vi "Turret Controller.vi"(8 "error in":errorcluster) -> ()   [LabVIEW 2015]
doc: "This VI executes continuously carrying out the current operation and responding to updates or new operations. It will often contain the timing or control code that is difficult to place directly in TeleOp. This VI generally opens all sensors and motors and isolates the rest of the robot code from knowing how the operations are carried out."
uses:
  Turret Setpoints.ctl
  Turret Operations.ctl
  <vilib>/Rock Robotics/WPI/CAN/TalonSRX/WPI_CANTalonSRX_APIControlMode.ctl
  <vilib>/Rock Robotics/WPI/CAN/TalonSRX/WPI_CANTalonSRX_APIFeedbackSelect.ctl
  <vilib>/Rock Robotics/WPI/CAN/TalonSRX/WPI_CANTalonSRX_Params.ctl
  <vilib>/Rock Robotics/WPI/MotorControl/WPI_MotorControlOpenCANTalonSRX.vi
  Framework/Robot Global Data.vi
  Vision/Vision Published Globals.vi
  Turret Published Globals.vi
  Support Code/navX Library v2/navX Library v2.lvlib
panel:
  out "Current\nCmd":string
  # "Tip: It may be helpful to observe inputs and sensor values.\nYou may also want to display tuning or debugging controls."
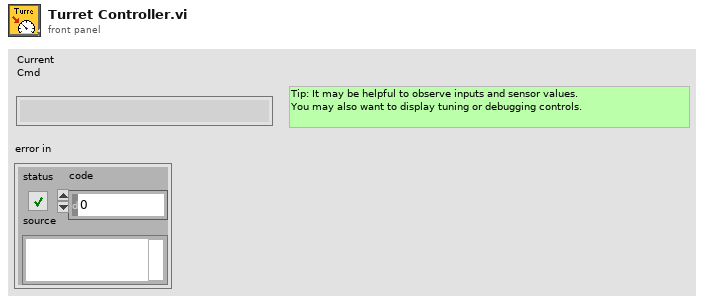
[diagram p1: front panel]
types:
  T1 = typedef "Turret Setpoints.ctl" = cluster{"Operation":T2, "Setpoint":dbl, "Duration":dbl}
  T2 = typedef "Turret Operations.ctl" = enum16{"Reserve", "Read Current", "Go to Angle (Turret Centric)", "Idle", "Go to Angle (Field Centric)", "Roaming", "Go to Angle", "Manual Control"}
  T3 = typedef "WPI_CANTalonSRX_APIFeedbackSelect.ctl" = enum16{"Digital Quadrature Encoder", "Analog Potentiometer", "Analog Encoder", "Count on Quad-A (Rising-Edge)", "Count on Quad-A (Falling-Edge)", "CTR Magnetic Enc (Absolute)", "CTR Magnetic Enc (Relative)", "Pulse Width"}
  T4 = typedef "WPI_CANTalonSRX_APIControlMode.ctl" = enum8{"Percent VBus", "Speed", "Position", "Slave", "Unchanged / Invalid", "Voltage Compensation", "Current", "Motion Profile"}
  T5 = typedef "WPI_MotorControlDeviceRef.ctl" = cluster{"DeviceStatus":errorcluster, "Type":T6, "PWM":cluster{"PWM Channel":T7, "DeadBand":T8}, "CAN":cluster{"Device Number":u8, "Control Mode":T9, "Semaphore":T10, "Max Vout":dbl, "TalonSRX Control Mode":T4}, "Invert":bool}
  T6 = typedef "WPI_MotorControlType.ctl" = enum16{"PWM", "CAN", "CANTalonSRX"}
  T7 = typedef "FPGA_DIOPWMChannel.ctl" = enum8{"PWM 0", "PWM 1", "PWM 2", "PWM 3", "PWM 4", "PWM 5", "PWM 6", "PWM 7", "PWM 8", "PWM 9", "PWM MXP 0", "PWM MXP 1", "PWM MXP 2", "PWM MXP 3", "PWM MXP 4", "PWM MXP 5", "PWM MXP 6", "PWM MXP 7", "PWM MXP 8", "PWM MXP 9", "Invalid"}
  T8 = typedef "WPI_PWMDeadband.ctl" = cluster{"Name":string, "maxPositivePwm":i32, "minPositivePwm":i32, "centerPwm":i32, "maxNegativePwm":i32, "minNegativePwm":i32, "angularRange":u16}
  T9 = typedef "WPI_CANJaguar_ControlMode.ctl" = enum8{"Percent VBus", "Current", "Speed", "Position", "Voltage"}
  T10 = typedef "Semaphore RefNum" = refnum<k1>
  T11 = typedef "navX Library v2.lvlib/Z900_navX_DeviceTypeDef.ctl" = cluster{"Interface":cluster{"Protocol":T12, "Update Rate (4Hz-60Hz)":u8, "navX Open TypeDef":variant}, "Notify Packet":refnum<notifier>, "Loop VI Refnum":refnum<vi>, "Ready to Close Occurrence Refnum":refnum<k4>}
  T12 = typedef "navX Library v2.lvlib/Z900_navX_ProtocolTypeDef.ctl" = enum16{"SERIAL", "I2C", "SPI"}
  T13 = typedef "WPI_CANTalonSRX_Params.ctl" = u8
  T14 = typedef "Command Status Info.ctl" = cluster{"Name":string, "Status":T15, "notifier out":T16}
  T15 = typedef "Completion Status.ctl" = enum16{"Successful", "Aborted", "Incomplete"}
  T16 = typedef "Completion Notifier.ctl" = refnum<notifier>
  T17 = cluster{"Default Command":T1, "Command Timing":cluster{"Start Time (ms)":u32, "Iterations":i32}, "Command Arguments":cluster{"Command Info":T14, "Description":string, "Default Command":T1, "notifier out":refnum<notifier>, "Subsystem Name":string}}
  T18 = cluster{"Yaw":dbl, "Roll":dbl, "Pitch":dbl, "Heading":dbl, "Fused Heading":dbl}
  T19 = typedef "WPI_CANTalonSRX_GlobalStatus.ctl" = cluster{"Applied Throttle":dbl, "Module Enabled":bool, "CAN Error":errorcluster, "Closed Loop Error":dbl, "Forward Limit Switch Closed":bool, "Reverse Limit Switch Closed":bool, "Sensor Position":dbl, "Sensor Velocity":dbl, "Current":dbl, "Sticky Fault - Over Temp":bool, "Sticky Fault - Under Voltage":bool, "Sticky Fault - Forward Limit":bool, "Sticky Fault - Reverse Limit":bool, "Sticky Fault - Forward Soft Limit":bool, "Sticky Fault - Reverse Soft Limit":bool, "Brake is Enabled":bool, "Encoder Position":dbl, "Encoder Velocity":dbl, "Encoder Index Count":dbl, "Encoder A Pin State":bool, "Encoder B Pin State":bool, "Encoder Index Pin State":bool, "Analog In":dbl, "Analog In Velocity":dbl, "Temperature (C)":dbl, "Battery Voltage":dbl, "Control 5 Is Supported":bool, "Current Profile Slot Select":dbl, "Pos Div 8":bool, "Vel Div 4":bool, "Pulse Width Position":i32, "Pulse Width Velocity":i32, "Pulse Width Rise To Rise (us)":i32, "Pulse Width Rise To Fall (us)":i32, "Mot Prof Active Is Under Run":bool, "Mot Prof Active Has Under Run":bool, "Mot Prof Active Is Last":bool, "Mot Prof Active Velocity Only":bool, "Mot Prof Active Is Valid":bool, "Mot Prof Buffer Is Full":bool, "Mot Prof Active Profile Slot Select":i32, "Mot Prof NextID":i32, "Mot Prof Count":i32, "Mot Prof Active Velocity":dbl, "Mot Prof Active Position":dbl, "Mot Prof Output Enable":i32}
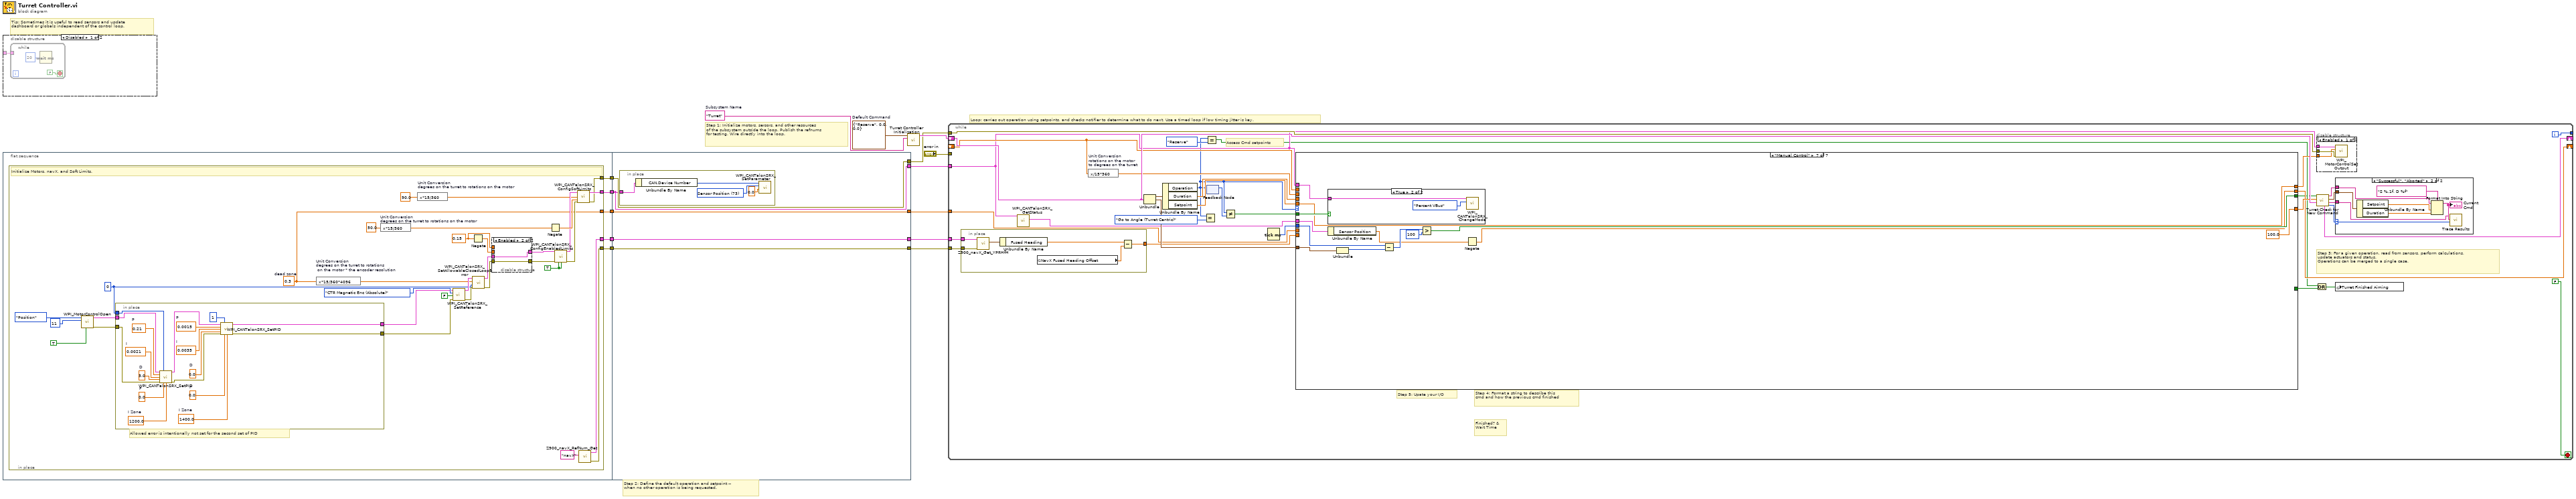
[diagram p0: block diagram]
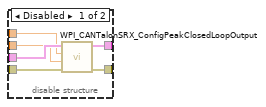
[diagram p2: hidden frame]
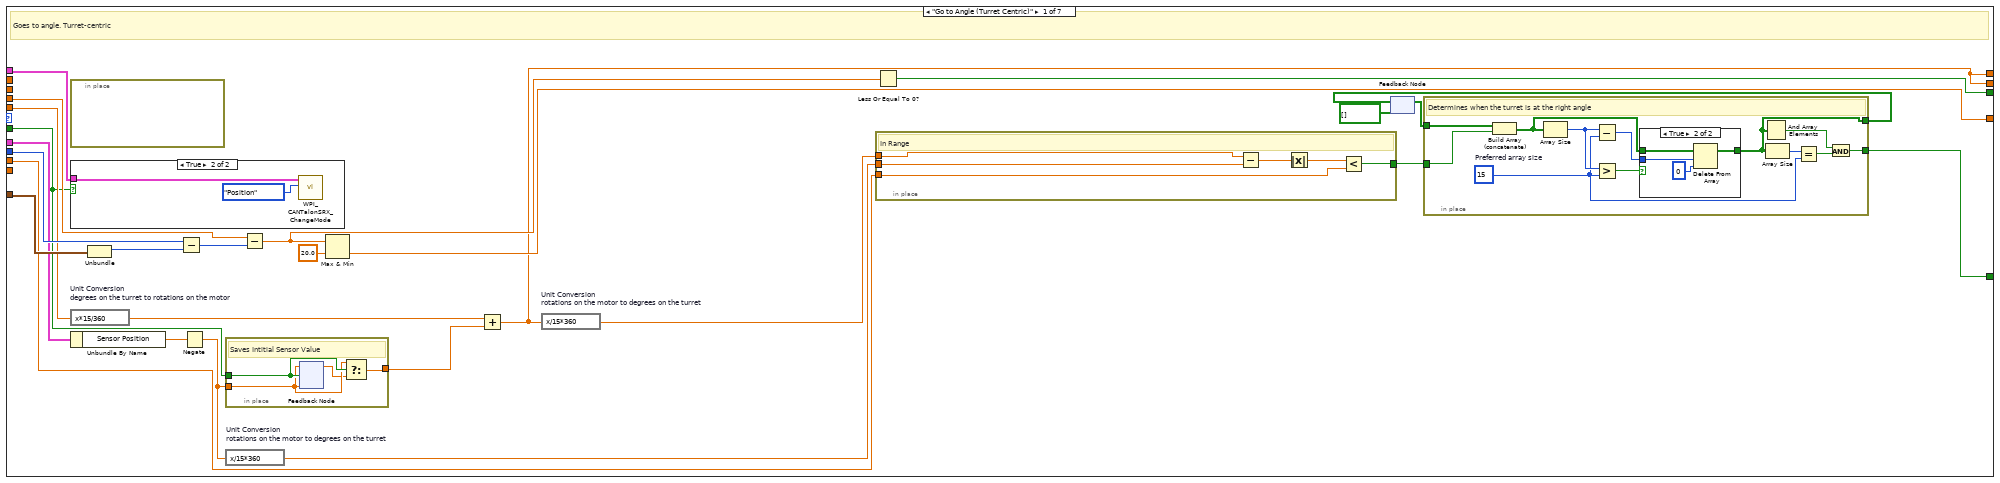
[diagram p6: hidden frame]
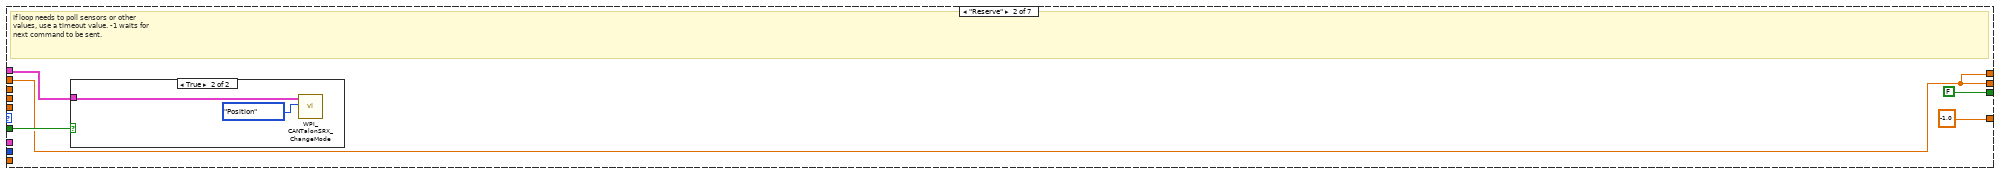
[diagram p9: hidden frame]
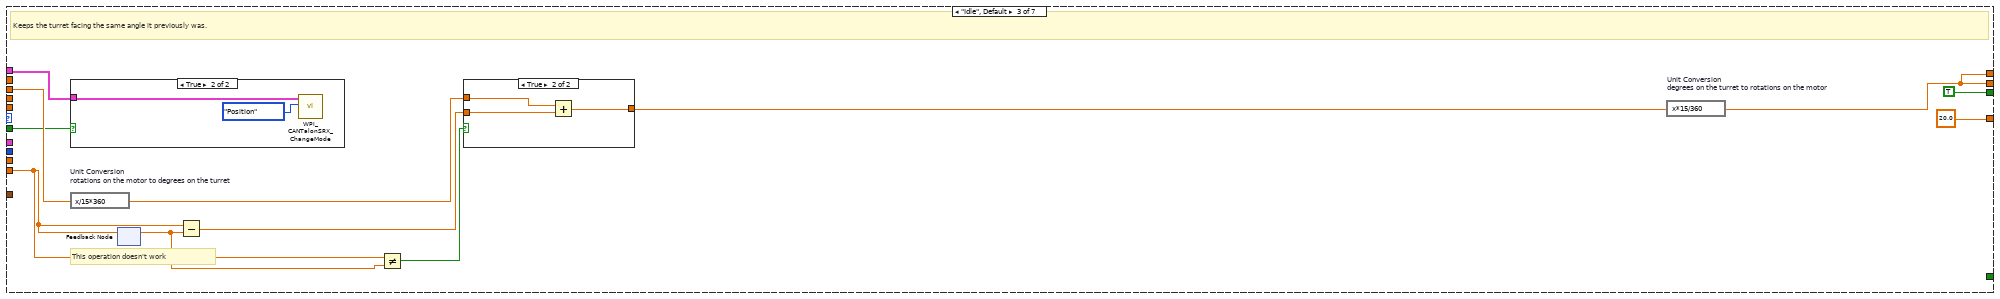
[diagram p11: hidden frame]
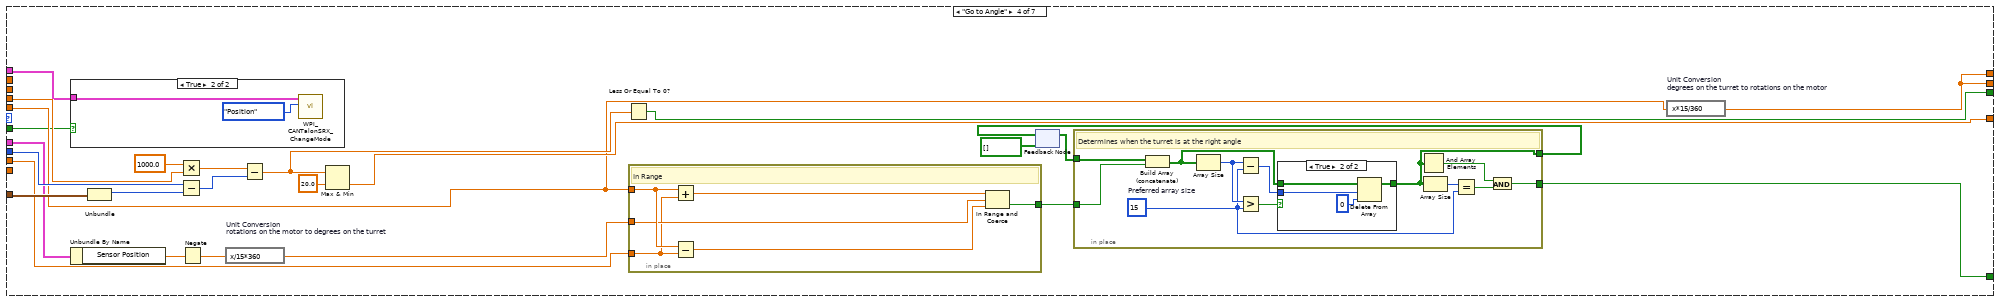
[diagram p14: hidden frame]
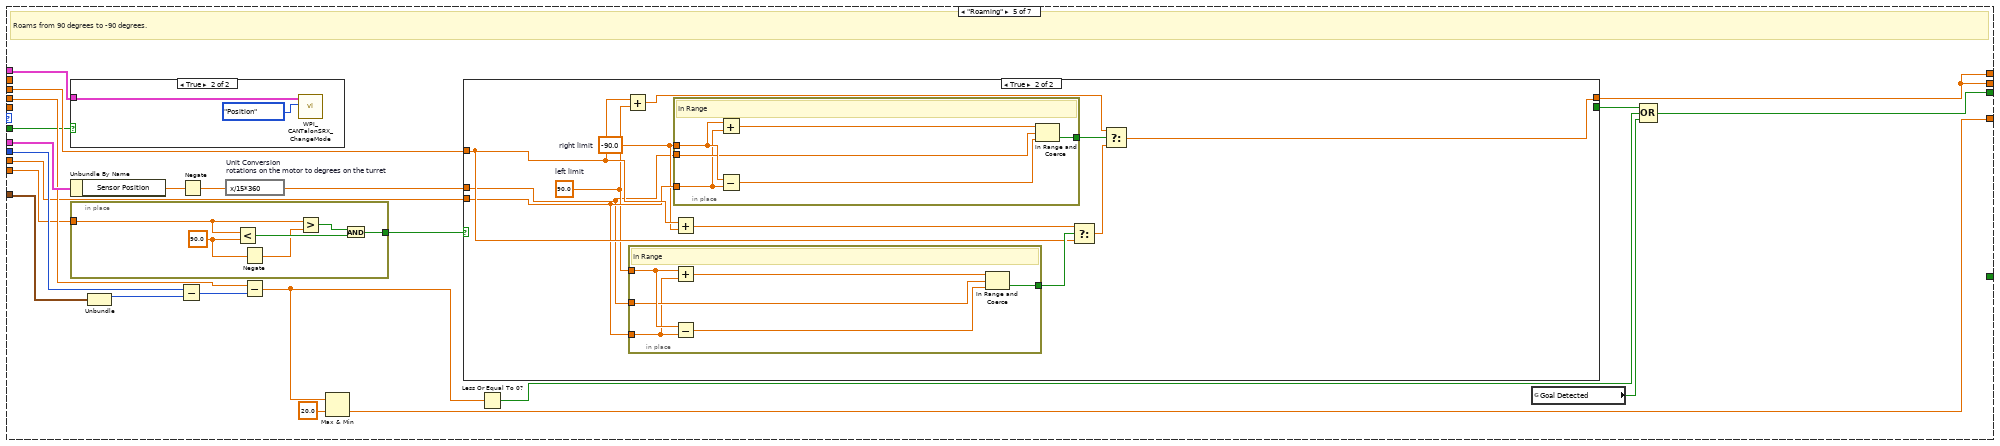
[diagram p17: hidden frame]
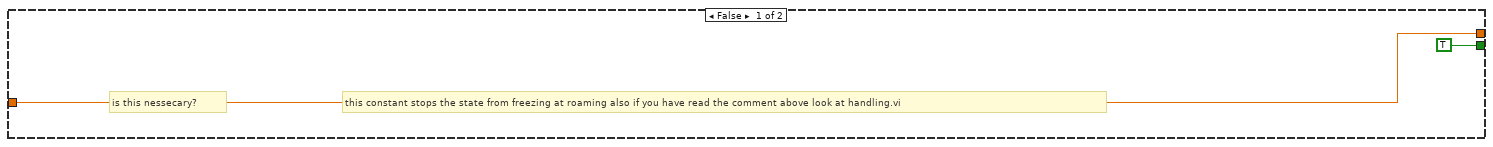
[diagram p19: hidden frame]
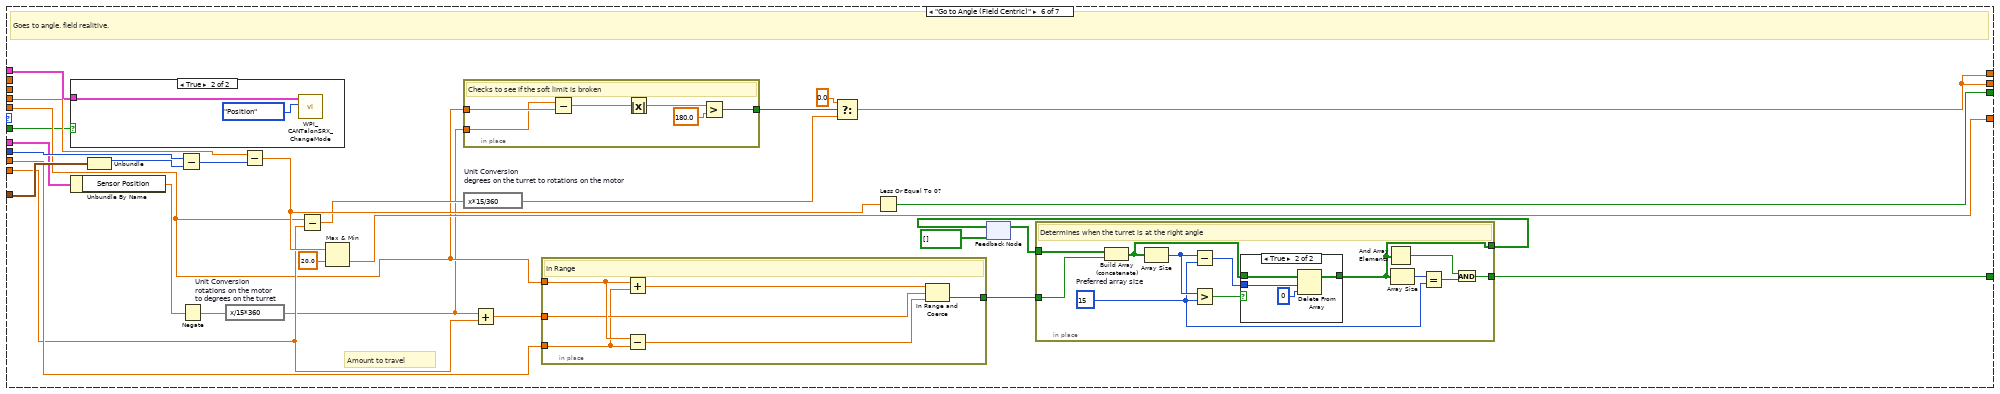
[diagram p20: hidden frame]
diagram:
  w11 = T1 {"Operation"=enum."Reserve", "Setpoint"=0.0, "Duration"=0.0}  # Default Command
  w12 = "Turret"  # Subsystem Name
  # "Step 2: Define the default operation and setpoint --\nwhen no other operation is being requested."
  # "Tip: Sometimes it is useful to read sensors and update\ndashboard or globals independent of the control loop."
  # "Step 1: Initialize motors, sersors, and other resources\nof the subsystem outside the loop. Publish the refnums\nfor testing. Wire directly into the loop."
  # "Loop: carries out operation using setpoints, and checks notifier to determine what to do next. Use a timed loop if low timing jitter is key."
  n1 = disable-structure shown="Disabled" {
    disable-tunnel: _ -> [w15 _]
    frame Disabled {
      n2 = while {
        tunnel: w15 -> [_]
        stop <- FALSE stop-if-true
        n3 = Wait (ms)(milliseconds to wait=u32 20) -> ()  [unwired: 1 out]
      }
    }
    frame Enabled {
    }
  }
  n4 = flat-sequence {
    tunnel: [w22] -> w5
    tunnel: [w21] -> w4
    tunnel: [w20] -> w3
    tunnel: [w19] -> w2
    tunnel: [w18] -> w1
    tunnel: [w83] -> w6
    tunnel: [w84] -> w7
    tunnel: [w85] -> w8
    tunnel: [w86] -> w9
    tunnel: [w82] -> w10
    tunnel: w5 -> [w82]
    tunnel: w4 -> [w86]
    tunnel: w3 -> [w85]
    tunnel: w2 -> [w84]
    tunnel: w1 -> [w83]
    frame #0 {
      n5 = in-place {
        in-place-border: [w48] -> w22
        in-place-border: [w47] -> w21
        in-place-border: [w45] -> w20
        in-place-border: [w44] -> w19
        in-place-border: [w27] -> w18
        w30 = 0.15
        w27 = 0.3  # dead zone
        w31 = u8 0 ("Parameter Slot")
        w34 = TRUE ("Forward Soft Limit Enable")
        # "Allowed error is intentionally not set for the second set of PID"
        # "Initialize Motors, navX, and Soft Limits."
        n6 = call-poly <vilib>:"WPI_MotorControlOpen.vi"("Invert"=TRUE, "Device Number"=11, "Control Mode"=WPI_CANTalonSRX_APIControlMode."Position") -> ("error out"=w52:errorcluster, "MotorControlDeviceRef"=w53:T5)  [unwired: 7 in]
        n7 = in-place {
          in-place-border: w53 -> [w81]
          in-place-border: w52 -> [w80]
          in-place-border: [w70] -> w51
          in-place-border: [w72] -> w25
          in-place-border: w31 -> [w74]
          w65 = 1400.0  # I Zone
          w66 = 0.0  # F
          w67 = 0.0  # D
          w68 = 0.0035  # I
          w69 = 0.0015  # P
          w75 = 1200.0  # I Zone
          w76 = 0.0  # F
          w77 = 3.0  # D
          w78 = 0.0021  # I
          w79 = 0.21  # P
          n8 = call <vilib>:"WPI_CANTalonSRX_SetPID.vi"("CAN Talon SRX Ref"=w81, "Parameter Slot"=w74, "P"=w79, "I"=w78, "D"=w77, "error in (no error)"=w80, "F"=w76, "I Zone"=w75) -> ("CAN Talon SRX Ref"=w73:T5, "error out"=w71:errorcluster)  [unwired: 6 in]
          n9 = call <vilib>:"WPI_CANTalonSRX_SetPID.vi"("CAN Talon SRX Ref"=w73, "Parameter Slot"=u8 1, "P"=w69, "I"=w68, "D"=w67, "error in (no error)"=w71, "F"=w66, "I Zone"=w65) -> ("CAN Talon SRX Ref"=w72:T5, "error out"=w70:errorcluster)  [unwired: 6 in]
        }
        n10 = expression code="x*15/360*4096" "Unit Conversion\ndegrees on the turret to rotations\n on the motor * the encoder resolution"(w27) -> (w26:dbl)
        n11 = expression code="x*15/360" "Unit Conversion\ndegrees on the turret to rotations on the motor"(50.0 ("Forward Limit Position")) -> (w42:dbl)
        n12 = expression code="x*15/360" "Unit Conversion\ndegrees on the turret to rotations on the motor"(90.0 ("Forward Limit Position")) -> (w23:dbl)
        n13 = call <vilib>:"WPI_CANTalonSRX_SetReference.vi"("error in (no error)"=w51, "Reverse Feedback Sensor"=FALSE, "Feedback Reference"=WPI_CANTalonSRX_APIFeedbackSelect."CTR Magnetic Enc (Absolute)", "CAN Talon SRX Ref"=w25) -> ("error out"=w40:errorcluster, "CAN Talon SRX Ref"=w39:T5)  [unwired: 6 in]
        n14 = Negate(x=w30) -> (-x=w29:dbl)
        n15 = call <vilib>:"WPI_CANTalonSRX_SetAllowableClosedLoopError.vi"("error in (no error)"=w40, "Parameter Slot"=w31, "Allowable Closed-Loop Error"=w26, "CAN Talon SRX Ref"=w39) -> ("error out"=w38:errorcluster, "CAN Talon SRX Ref"=w37:T5)  [unwired: 6 in]
        n16 = disable-structure shown="Enabled" {
          disable-tunnel: w38 -> [w61 w62]
          disable-tunnel: w37 -> [w60 w63]
          disable-tunnel: [w59 w63] -> w36
          disable-tunnel: [w58 w62] -> w35
          disable-tunnel: w30 -> [w57 _]
          disable-tunnel: w29 -> [w56 _]
          frame Disabled {
            n17 = call <vilib>:"WPI_CANTalonSRX_ConfigPeakClosedLoopOutput.vi"("error in (no error)"=w61, "Reverse Peak Output"=w56, "Forward Peak Output"=w57, "CAN Talon SRX Ref"=w60) -> ("error out"=w58:errorcluster, "CAN Talon SRX Ref"=w59:T5)  [unwired: 6 in]
          }
          frame Enabled {
          }
        }
        n18 = Negate(x=w42) -> (-x=w41:dbl)
        n19 = call <vilib>:"WPI_CANTalonSRX_ConfigEnabledLimits.vi"("CAN Talon SRX Ref"=w36, "error in (no error)"=w35, "Forward Soft Limit Enable"=w34, "Reverse Soft Limit Enable"=w34) -> ("CAN Talon SRX Ref"=w32:T5, "error out"=w33:errorcluster)  [unwired: 10 in]
        n20 = call <vilib>:"WPI_CANTalonSRX_ConfigSoftLimits.vi"("CAN Talon SRX Ref"=w32, "Forward Limit Position"=w23, "Reverse Limit Position"=w41, "error in (no error)"=w33) -> ("CAN Talon SRX Ref"=w48:T5, "error out"=w47:errorcluster)  [unwired: 10 in]
        n21 = call "Z900_navX_RefNum_Get.vi"("refnum name"="navX") -> ("error out"=w45:errorcluster, "navX Device"=w44:T11)  [unwired: 9 in]
      }
    }
    frame #1 {
      n22 = in-place {
        in-place-border: w82 -> [w90]
        w88 = T13 73 items=["Slot 0 - P"=1, "Slot 0 - I"=2, "Slot 0 - D"=3, "Slot 0 - F"=4, "Slot 0 - I Zone"=5, "Slot 0 - Ramp Rate"=6, "Slot 1 - P"=11, "Slot 1 - I"=12, "Slot 1 - D"=13, "Slot 1 - F"=14, "Slot 1 - I Zone"=15, "Slot 1 - Ramp Rate"=16, "Soft Limit - Forward"=21, "Soft Limit - Reverse"=22, "On Boot - Brake Mode"=31, "On Boot - Limit Normally Closed - Forward"=32, "On Boot - Limit Normally Closed - Reverse"=33, "On Boot - Limit Disabled - Forward"=34, "On Boot - Limit Disabled - Reverse"=35, "Fault - Over Temp"=41, "Fault - Under Voltage"=42, "Fault - Forward Limit"=43, "Fault - Reverse Limit"=44, "Fault - Hardware Failure"=45, "Fault - Forward Soft Limit"=46, "Fault - Reverse Soft Limit"=47, "Sticky Fault - Over Temp"=48, "Sticky Fault - Under Voltage"=49, "Sticky Fault - Forward Limit"=50, "Sticky Fault - Reverse Limit"=51, "Sticky Fault - Forward Soft Limit"=52, "Sticky Fault - Reverse Soft Limit"=53, "Applied Throttle"=61, "Closed-Loop Error"=62, "Select Feedback Device"=63, "Reverse Closed-Loop Output"=64, "Mode Select"=65, "Profile Slot Select"=66, "Ramp Throttle"=67, "Reverse Feedback Sensor"=68, "Limit Switch Enabled"=69, "Limit Switch Closed - Forward"=70, "Limit Switch Closed - Reverse"=71, "Sensor Position"=73, "Sensor Velocity"=74, "Current"=75, "Brake is Enabled"=76, "Encoder Position"=77, "Encoder Velocity"=78, "Encoder Index Rise Events"=79, "Encoder A Pin State"=80, "Encoder B Pin State"=81, "Encoder Index Pin State"=82, "Analog In with Overflow"=83, "Analog In Velocity"=84, "Temperature"=85, "Battery Voltage"=86, "Reset Count"=87, "Reset Flags"=88, "Firmware Version"=89, "Settings Changed"=90] ("Parameter")
        n23 = Unbundle By Name(w90) -> ("CAN.Device Number"=w89:u8)
        n24 = call <vilib>:"WPI_CANTalonSRX_SetParameter.vi"("Value"=0.0, "Parameter"=w88, "Device ID (0)"=w89) -> ()  [unwired: 7 in, 2 out]
      }
    }
  }
  n25 = call "Turret Controller Initialization.vi"("Subsystem Name"=w12, "Default Command"=w11) -> ("Command Info"=w13:T17)  [unwired: 9 in]
  n26 = while {
    shift-right: [w117] -> _
    shift-left: w13 -> [w118]
    tunnel: [w123] -> _
    tunnel: "error in" -> [_]
    tunnel: w10 -> [w99]
    tunnel: w9 -> [w109]
    tunnel: w8 -> [w110]
    tunnel: w7 -> [w111]
    tunnel: w6 -> [w107]
    shift-right: [w105] -> _
    shift-left: _ -> [w100]
    i -> [w123]
    stop <- FALSE stop-if-true
    # "Step 5: Upate your I/O"
    # "Step 4: Format a string to describe this\ncmd and how the previous cmd finished"
    # "Access Cmd setpoints"
    # "Finished? &\nWait Time"
    # "Step 3: For a given operation, read from sensors, perform calculations,\nupdate actuators and status.\nOperations can be merged to a single case."
    n27 = in-place {
      in-place-border: w111 -> [w130]
      in-place-border: w110 -> [w129]
      in-place-border: [w126] -> w106
      n28 = call "Z900_navX_Get_YPRHfH.vi"("error in (no error)"=w129, "navX Device"=w130) -> ("YRPHfH"=w125:T18)  [unwired: 6 in, 3 out]
      n29 = Unbundle By Name(w125) -> ("Fused Heading"=w128:dbl)
      n30 = global read "Robot Global Data.vi" "NavX Fused Heading Offset"() -> (w127:dbl)
      n31 = Subtract(x=w128, y=w127) -> (x-y=w126:dbl)
    }
    n32 = call <vilib>:"WPI_CANTalonSRX_GetStatus.vi"("CAN Talon SRX Ref"=w99) -> ("Talon SRX Status"=w108:T19)  [unwired: 8 in, 2 out]
    n33 = expression code="x/15*360" "Unit Conversion\nrotations on the motor to degrees on the turret"(w100) -> (w103:dbl)
    n34 = Unbundle(w118) -> ("Default Command"=w122:T1, "Command Timing"=w120:cluster{"Start Time (ms)":u32, "Iterations":i32})  [unwired: 1 out]
    n35 = Unbundle By Name(w122) -> ("Operation"=w93:T2, "Duration"=w104:dbl, "Setpoint"=w119:dbl)
    n36 = Equal?(x=w93, y=Turret_Operations."Go to Angle (Turret Centric)") -> ()  [unwired: 1 out]
    n37 = Equal?(x=w93, y=Turret_Operations."Reserve") -> (x = y?=w95:bool)
    n38 = feedback #1() -> (w102:T2)  [unwired: 1 in]
    n39 = feedback-in #1(w93) -> ()
    n40 = Not Equal?(x=w93, y=w102) -> (x != y?=w101:bool)
    n41 = Tick Count (ms)() -> (millisecond timer value=w121:u32)
    n42 = case shown="\"Manual Control\"" w93 {
      tunnel: [w158 -1.0 20.0 w240 w279 w349 100.0] -> w116
      tunnel: [w142 FALSE ("ignore previous (F)") TRUE ("ignore previous (F)") w223 w280 w329 w395] -> w94
      tunnel: w120 -> [w166 _ _ w243 w285 w354 w397]
      tunnel: w104 -> [w159 _ _ w238 w282 w350 _]
      tunnel: w121 -> [w165 _ _ w242 w283 w353 w396]
      tunnel: w119 -> [w156 _ _ w234 _ w343 w389]
      tunnel: w108 -> [w163 _ _ w236 w286 w338 w391]
      tunnel: [w149 w197 w204 w229 w273 w335 w388] -> w105
      tunnel: w107 -> [w164 _ _ w235 w281 w345 _]
      tunnel: w106 -> [_ _ w209 _ w277 w344 _]
      tunnel: w103 -> [_ _ w207 _ w284 _ _]
      tunnel: w100 -> [_ w197 _ _ _ _ _]
      tunnel: w101 -> [w150 w198 w205 w231 w274 w336 w399]
      tunnel: w99 -> [w151 w199 w206 w230 w275 w337 w400]
      tunnel: [w149 w197 w204 w229 w273 w335 w389] -> w98
      tunnel: [w143 _ _ w222 _ w328 _] -> w91
      frame "Go to Angle (Turret Centric)" {
        # "Goes to angle. Turret-centric"
        n43 = in-place {
        }
        n44 = case shown="True" w150 {
          tunnel: w151 -> [_ w186]
          frame False {
          }
          frame True {
            n45 = call <vilib>:"WPI_CANTalonSRX_ChangeMode.vi"("Control Mode"=WPI_CANTalonSRX_APIControlMode."Position", "CAN Talon SRX Ref"=w186) -> ()  [unwired: 8 in, 2 out]
          }
        }
        n46 = expression code="x*15/360" "Unit Conversion\ndegrees on the turret to rotations on the motor"(w156) -> (w155:dbl)
        n47 = Unbundle By Name(w163) -> ("Sensor Position"=w153:dbl)
        n48 = Unbundle(w166) -> ("Start Time (ms)"=w167:u32)  [unwired: 1 out]
        n49 = Subtract(x=w165, y=w167) -> (x-y=w162:u32)
        n50 = Negate(x=w153) -> (-x=w148:dbl)
        n51 = in-place {
          in-place-border: w150 -> [w190]
          in-place-border: w148 -> [w189]
          in-place-border: [w187] -> w152
          # "Saves Intitial Sensor Value"
          n52 = feedback #2(w189) -> (w188:dbl)
          n53 = feedback-in #2(w189, w190) -> ()
          n54 = Select(t=w189, s=w190, f=w188) -> (s? t:f=w187:dbl)
        }
        n55 = expression code="x/15*360" "Unit Conversion\nrotations on the motor to degrees on the turret"(w148) -> (w160:dbl)
        n56 = Subtract(x=w159, y=w162) -> (x-y=w157:dbl)
        n57 = Max & Min(x=w157, y=20.0) -> (min(x,y)=w158:dbl)  [unwired: 1 out]
        n58 = Add(x=w155, y=w152) -> (x+y=w149:dbl)
        n59 = expression code="x/15*360" "Unit Conversion\nrotations on the motor to degrees on the turret"(w149) -> (w154:dbl)
        n60 = in-place {
          in-place-border: [w191] -> w144
          in-place-border: w154 -> [w196]
          in-place-border: w160 -> [w195]
          in-place-border: w164 -> [w192]
          # "In Range"
          n61 = Subtract(x=w196, y=w195) -> (x-y=w194:dbl)
          n62 = Absolute Value(x=w194) -> (abs(x)=w193:dbl)
          n63 = Less?(x=w193, y=w192) -> (x < y?=w191:bool)
        }
        n64 = Less Or Equal To 0?(x=w157) -> (x <= 0?=w142:bool)
        n65 = feedback #3(bool[] []) -> (w147:bool[])
        n66 = in-place {
          in-place-border: w147 -> [w179]
          in-place-border: [w172] -> w146
          in-place-border: [w169] -> w143
          in-place-border: w144 -> [w168]
          w173 = 15  # Preferred array size
          # "Determines when the turret is at the right angle"
          n67 = Build Array (concatenate)(w179, w168) -> (w178:bool[])
          n68 = Array Size(array=w178) -> (size(s)=w176:i32)
          n69 = Subtract(x=w176, y=w173) -> (x-y=w175:i32)
          n70 = Greater?(x=w176, y=w173) -> (0:w177:bool)
          n71 = case shown="True" w177 {
            tunnel: w178 -> [w180 w184]
            tunnel: [w180 w183] -> w172
            tunnel: w175 -> [_ w182]
            frame False {
            }
            frame True {
              n72 = Delete From Array(array=w184, length=w182, index=0) -> (array with subset deleted=w183:bool[])  [unwired: 1 out]
            }
          }
          n73 = And Array Elements(Boolean array=w172) -> (logical AND=w174:bool)
          n74 = Array Size(array=w172) -> (size(s)=w170:i32)
          n75 = Equal?(x=w170, y=w173) -> (x = y?=w171:bool)
          n76 = And(x=w174, y=w171) -> (x .and. y?=w169:bool)
        }
        n77 = feedback-in #3(w146) -> ()
      }
      frame "Reserve" {
        # "If loop needs to poll sensors or other\nvalues, use a timeout value. -1 waits for\nnext command to be sent."
        n78 = case shown="True" w198 {
          tunnel: w199 -> [_ w203]
          frame False {
          }
          frame True {
            n79 = call <vilib>:"WPI_CANTalonSRX_ChangeMode.vi"("Control Mode"=WPI_CANTalonSRX_APIControlMode."Position", "CAN Talon SRX Ref"=w203) -> ()  [unwired: 8 in, 2 out]
          }
        }
      }
      frame "Idle", Default {
        # "This operation doesn't work"
        # "Keeps the turret facing the same angle it previously was."
        n80 = case shown="True" w205 {
          tunnel: w206 -> [_ w217]
          frame False {
          }
          frame True {
            n81 = call <vilib>:"WPI_CANTalonSRX_ChangeMode.vi"("Control Mode"=WPI_CANTalonSRX_APIControlMode."Position", "CAN Talon SRX Ref"=w217) -> ()  [unwired: 8 in, 2 out]
          }
        }
        n82 = expression code="x/15*360" "Unit Conversion\nrotations on the motor to degrees on the turret"(w207) -> (w210:dbl)
        n83 = feedback-in #4(w209) -> ()
        n84 = feedback #4() -> (w212:dbl)  [unwired: 1 in]
        n85 = Subtract(x=w209, y=w212) -> (x-y=w211:dbl)
        n86 = Not Equal?(x=w209, y=w212) -> (x != y?=w213:bool)
        n87 = case shown="True" w213 {
          tunnel: w211 -> [_ w219]
          tunnel: w210 -> [w218 w221]
          tunnel: [w218 w220] -> w208
          frame False {
          }
          frame True {
            n88 = Add(x=w221, y=w219) -> (x+y=w220:dbl)
          }
        }
        n89 = expression code="x*15/360" "Unit Conversion\ndegrees on the turret to rotations on the motor"(w208) -> (w204:dbl)
      }
      frame "Go to Angle" {
        n90 = case shown="True" w231 {
          tunnel: w230 -> [_ w265]
          frame False {
          }
          frame True {
            n91 = call <vilib>:"WPI_CANTalonSRX_ChangeMode.vi"("Control Mode"=WPI_CANTalonSRX_APIControlMode."Position", "CAN Talon SRX Ref"=w265) -> ()  [unwired: 8 in, 2 out]
          }
        }
        n92 = Unbundle By Name(w236) -> ("Sensor Position"=w233:dbl)
        n93 = Unbundle(w243) -> ("Start Time (ms)"=w244:u32)  [unwired: 1 out]
        n94 = Multiply(x=1000.0, y=w238) -> (x*y=w237:dbl)
        n95 = Subtract(x=w242, y=w244) -> (x-y=w246:u32)
        n96 = Negate(x=w233) -> (-x=w228:dbl)
        n97 = expression code="x/15*360" "Unit Conversion\nrotations on the motor to degrees on the turret"(w228) -> (w232:dbl)
        n98 = Subtract(x=w237, y=w246) -> (x-y=w241:dbl)
        n99 = Max & Min(x=w241, y=20.0) -> (min(x,y)=w240:dbl)  [unwired: 1 out]
        n100 = Less Or Equal To 0?(x=w241) -> (x <= 0?=w223:bool)
        n101 = in-place {
          in-place-border: [w271] -> w224
          in-place-border: w234 -> [w268]
          in-place-border: w232 -> [w267]
          in-place-border: w235 -> [w266]
          # "In Range"
          n102 = Add(x=w268, y=w266) -> (x+y=w270:dbl)
          n103 = Subtract(x=w268, y=w266) -> (x-y=w269:dbl)
          n104 = In Range and Coerce(upper limit=w270, x=w267, lower limit=w269) -> (In Range?=w271:bool)  [unwired: 1 out]
        }
        n105 = feedback #5(bool[] []) -> (w227:bool[])
        n106 = in-place {
          in-place-border: w227 -> [w258]
          in-place-border: [w251] -> w226
          in-place-border: [w248] -> w222
          in-place-border: w224 -> [w247]
          w252 = 15  # Preferred array size
          # "Determines when the turret is at the right angle"
          n107 = Build Array (concatenate)(w258, w247) -> (w257:bool[])
          n108 = Array Size(array=w257) -> (size(s)=w255:i32)
          n109 = Subtract(x=w255, y=w252) -> (x-y=w254:i32)
          n110 = Greater?(x=w255, y=w252) -> (0:w256:bool)
          n111 = case shown="True" w256 {
            tunnel: w257 -> [w259 w263]
            tunnel: [w259 w262] -> w251
            tunnel: w254 -> [_ w261]
            frame False {
            }
            frame True {
              n112 = Delete From Array(array=w263, length=w261, index=0) -> (array with subset deleted=w262:bool[])  [unwired: 1 out]
            }
          }
          n113 = And Array Elements(Boolean array=w251) -> (logical AND=w253:bool)
          n114 = Array Size(array=w251) -> (size(s)=w249:i32)
          n115 = Equal?(x=w249, y=w252) -> (x = y?=w250:bool)
          n116 = And(x=w253, y=w250) -> (x .and. y?=w248:bool)
        }
        n117 = feedback-in #5(w226) -> ()
        n118 = expression code="x*15/360" "Unit Conversion\ndegrees on the turret to rotations on the motor"(w234) -> (w229:dbl)
      }
      frame "Roaming" {
        # "Roams from 90 degrees to -90 degrees."
        n119 = case shown="True" w274 {
          tunnel: w275 -> [_ w296]
          frame False {
          }
          frame True {
            n120 = call <vilib>:"WPI_CANTalonSRX_ChangeMode.vi"("Control Mode"=WPI_CANTalonSRX_APIControlMode."Position", "CAN Talon SRX Ref"=w296) -> ()  [unwired: 8 in, 2 out]
          }
        }
        n121 = Unbundle By Name(w286) -> ("Sensor Position"=w293:dbl)
        n122 = in-place {
          in-place-border: [w300] -> w278
          in-place-border: w277 -> [w297]
          w299 = 90.0
          n123 = Less?(x=w297, y=w299) -> (x < y?=w302:bool)
          n124 = Negate(x=w299) -> (-x=w298:dbl)
          n125 = Greater?(x=w297, y=w298) -> (0:w301:bool)
          n126 = And(x=w301, y=w302) -> (x .and. y?=w300:bool)
        }
        n127 = Unbundle(w285) -> ("Start Time (ms)"=w289:u32)  [unwired: 1 out]
        n128 = Subtract(x=w283, y=w289) -> (x-y=w288:u32)
        n129 = Negate(x=w293) -> (-x=w272:dbl)
        n130 = expression code="x/15*360" "Unit Conversion\nrotations on the motor to degrees on the turret"(w272) -> (w292:dbl)
        n131 = Subtract(x=w282, y=w288) -> (x-y=w287:dbl)
        n132 = Max & Min(x=w287, y=20.0) -> (min(x,y)=w279:dbl)  [unwired: 1 out]
        n133 = case shown="True" w278 {
          tunnel: w292 -> [_ w305]
          tunnel: w284 -> [w304 w310]
          tunnel: w281 -> [_ w309]
          tunnel: [w304 w308] -> w273
          tunnel: [TRUE _] -> w276
          frame False {
            # "this constant stops the state from freezing at roaming also if you have read the comment above look at handling.vi"
            # "is this nessecary?"
          }
          frame True {
            w307 = 90.0  # left limit
            w306 = -90.0  # right limit
            n134 = Add(x=w310, y=w307) -> (x+y=w313:dbl)
            n135 = in-place {
              in-place-border: [w327] -> w312
              in-place-border: w307 -> [w324]
              in-place-border: w305 -> [w323]
              in-place-border: w309 -> [w322]
              # "In Range"
              n136 = Add(x=w324, y=w322) -> (x+y=w326:dbl)
              n137 = Subtract(x=w324, y=w322) -> (x-y=w325:dbl)
              n138 = In Range and Coerce(upper limit=w326, x=w323, lower limit=w325) -> (In Range?=w327:bool)  [unwired: 1 out]
            }
            n139 = in-place {
              in-place-border: [w321] -> w315
              in-place-border: w306 -> [w318]
              in-place-border: w305 -> [w317]
              in-place-border: w309 -> [w316]
              # "In Range"
              n140 = Add(x=w318, y=w316) -> (x+y=w320:dbl)
              n141 = Subtract(x=w318, y=w316) -> (x-y=w319:dbl)
              n142 = In Range and Coerce(upper limit=w320, x=w317, lower limit=w319) -> (In Range?=w321:bool)  [unwired: 1 out]
            }
            n143 = Add(x=w310, y=w306) -> (x+y=w311:dbl)
            n144 = Select(t=w311, s=w312, f=w310) -> (s? t:f=w314:dbl)
            n145 = Select(t=w313, s=w315, f=w314) -> (s? t:f=w308:dbl)
          }
        }
        n146 = Less Or Equal To 0?(x=w287) -> (x <= 0?=w290:bool)
        n147 = global read "Vision Published Globals.vi" "Goal Detected"() -> (w294:bool)
        n148 = Compound Arithmetic op=OR(w276, w290, w294) -> (w280:bool)
      }
      frame "Go to Angle (Field Centric)" {
        # "Amount to travel"
        # "Goes to angle. field realitive."
        n149 = case shown="True" w336 {
          tunnel: w337 -> [_ w375]
          frame False {
          }
          frame True {
            n150 = call <vilib>:"WPI_CANTalonSRX_ChangeMode.vi"("Control Mode"=WPI_CANTalonSRX_APIControlMode."Position", "CAN Talon SRX Ref"=w375) -> ()  [unwired: 8 in, 2 out]
          }
        }
        n151 = Unbundle By Name(w338) -> ("Sensor Position"=w346:dbl)
        n152 = Unbundle(w354) -> ("Start Time (ms)"=w355:u32)  [unwired: 1 out]
        n153 = Subtract(x=w353, y=w355) -> (x-y=w351:u32)
        n154 = Negate(x=w346) -> (-x=w334:dbl)
        n155 = expression code="x/15*360" "Unit Conversion\nrotations on the motor to degrees on the turret"(w334) -> (w342:dbl)
        n156 = Subtract(x=w350, y=w351) -> (x-y=w348:dbl)
        n157 = Subtract(x=w343, y=w344) -> (x-y=w347:dbl)
        n158 = Max & Min(x=w348, y=20.0) -> (min(x,y)=w349:dbl)  [unwired: 1 out]
        n159 = in-place {
          in-place-border: w343 -> [w381]
          in-place-border: w342 -> [w380]
          in-place-border: [w376] -> w341
          # "Checks to see if the soft limit is broken"
          n160 = Subtract(x=w380, y=w381) -> (x-y=w379:dbl)
          n161 = Absolute Value(x=w379) -> (abs(x)=w378:dbl)
          n162 = Greater?(x=w378, y=180.0) -> (0:w376:bool)
        }
        n163 = expression code="x*15/360" "Unit Conversion\ndegrees on the turret to rotations on the motor"(w347) -> (w340:dbl)
        n164 = Add(x=w342, y=w344) -> (x+y=w356:dbl)
        n165 = in-place {
          in-place-border: [w387] -> w330
          in-place-border: w343 -> [w384]
          in-place-border: w356 -> [w383]
          in-place-border: w345 -> [w382]
          # "In Range"
          n166 = Add(x=w384, y=w382) -> (x+y=w386:dbl)
          n167 = Subtract(x=w384, y=w382) -> (x-y=w385:dbl)
          n168 = In Range and Coerce(upper limit=w386, x=w383, lower limit=w385) -> (In Range?=w387:bool)  [unwired: 1 out]
        }
        n169 = Select(t=0.0, s=w341, f=w340) -> (s? t:f=w335:dbl)
        n170 = Less Or Equal To 0?(x=w348) -> (x <= 0?=w329:bool)
        n171 = feedback #6(bool[] []) -> (w333:bool[])
        n172 = in-place {
          in-place-border: w333 -> [w368]
          in-place-border: [w361] -> w332
          in-place-border: [w358] -> w328
          in-place-border: w330 -> [w357]
          w362 = 15  # Preferred array size
          # "Determines when the turret is at the right angle"
          n173 = Build Array (concatenate)(w368, w357) -> (w367:bool[])
          n174 = Array Size(array=w367) -> (size(s)=w365:i32)
          n175 = Subtract(x=w365, y=w362) -> (x-y=w364:i32)
          n176 = Greater?(x=w365, y=w362) -> (0:w366:bool)
          n177 = case shown="True" w366 {
            tunnel: w367 -> [w369 w373]
            tunnel: [w369 w372] -> w361
            tunnel: w364 -> [_ w371]
            frame False {
            }
            frame True {
              n178 = Delete From Array(array=w373, length=w371, index=0) -> (array with subset deleted=w372:bool[])  [unwired: 1 out]
            }
          }
          n179 = And Array Elements(Boolean array=w361) -> (logical AND=w363:bool)
          n180 = Array Size(array=w361) -> (size(s)=w359:i32)
          n181 = Equal?(x=w359, y=w362) -> (x = y?=w360:bool)
          n182 = And(x=w363, y=w360) -> (x .and. y?=w358:bool)
        }
        n183 = feedback-in #6(w332) -> ()
      }
      frame "Manual Control" {
        n184 = case shown="True" w399 {
          tunnel: w400 -> [_ w402]
          frame False {
          }
          frame True {
            n185 = call <vilib>:"WPI_CANTalonSRX_ChangeMode.vi"("Control Mode"=WPI_CANTalonSRX_APIControlMode."Percent VBus", "CAN Talon SRX Ref"=w402) -> ()  [unwired: 8 in, 2 out]
          }
        }
        n186 = Unbundle By Name(w391) -> ("Sensor Position"=w390:dbl)
        n187 = Unbundle(w397) -> ("Start Time (ms)"=w398:u32)  [unwired: 1 out]
        n188 = Subtract(x=w396, y=w398) -> (x-y=w394:u32)
        n189 = Greater?(x=w394, y=u32 100) -> (0:w395:bool)
        n190 = Negate(x=w390) -> (-x=w388:dbl)
      }
    }
    n191 = Or(x=w95, y=w91) -> (x .or. y?=w96:bool)
    n192 = disable-structure shown="Enabled" {
      disable-tunnel: w109 -> [w133 _]
      disable-tunnel: w99 -> [w132 _]
      disable-tunnel: w98 -> [w131 _]
      frame Enabled {
        n193 = call <vilib>:"WPI_MotorControlSetOutput.vi"("error in (no error)"=w133, "Output"=w131, "MotorControlDevRef"=w132) -> ()  [unwired: 6 in, 3 out]
      }
      frame Disabled {
      }
    }
    n194 = call "Turret Check for New Command.vi"("Current Command"=w118, "Wait time (ms)"=w116, "Finished?"=w94) -> ("Completion"=w112:T15, "Subsystem Name"=w113:string, "Current Command"=w114:T1, "Initial Trace String"=w115:string, "NextCommand"=w117:T17)  [unwired: 4 in]
    n195 = case shown="\"Successful\", \"Aborted\"" w112 {
      selector: w112 -> [_ w141]
      tunnel: w115 -> [_ w137]
      tunnel: w114 -> [_ w138]
      tunnel: w113 -> [_ w134]
      frame "Incomplete", Default {
        # "Continuing current command"
      }
      frame "Successful", "Aborted" {
        # "Report and setup for next command"
        n196 = Unbundle By Name(w138) -> ("Setpoint"=w140:dbl, "Duration"=w135:dbl)
        n197 = Format Into String(format string="S %.1f, D %f", initial string=w137, w140, w135) -> (resulting string=w136:string)  [unwired: 1 in, 1 out]
        "Current\nCmd" <- w136
        n198 = call <vilib>:"Trace Results.vi"("Status of previous command"=w141, "Description"=w136, "Subsystem"=w134) -> ()  [unwired: 9 in]
      }
    }
    n199 = global write "Turret Published Globals.vi" "Turret Finished Aiming"(w96) -> ()
  }
